vi "G#Object_Deserialize.vi"(0 "reference in":refnum<class "G#Object.lvclass">, 1 "as xml (F)":bool, 2 "serialized object":string, 3 "class attributes (F)":bool, 4 "object id":u32[](array[numeric]), 5 "error in (no error)":errorcluster, 7 "include aggregates (T)":bool=TRUE) -> (14 "reference out":refnum<class "G#Object.lvclass">, 18 "object id out":u32[](array[numeric]), 19 "error out":errorcluster)   [LabVIEW 2020, in "G#Object.lvclass"]
doc: "Deserialize an object from a binary or XML string. \n\nNotice: Deserialization of aggregated objects is not supported by XML."
uses:
  G#Object.lvclass
  utils/G#Object_State.ctl
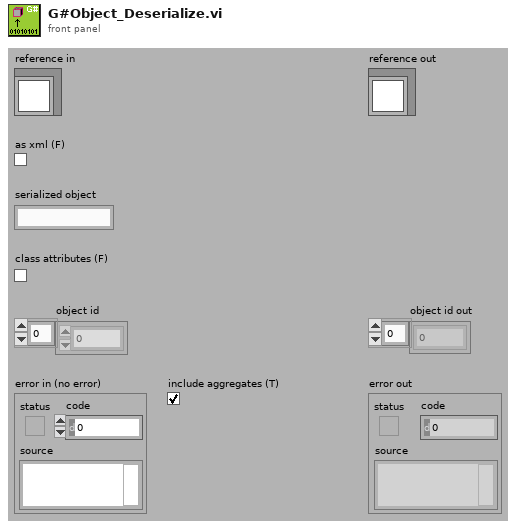
[diagram p1: front panel]
types:
  T1 = typedef "G#Object.lvclass/G#Object_State.ctl" = enum16{"Clear", "Create", "Delete", "Get class attributes", "Class hierarchy", "Get attribute value", "Set attribute value"}
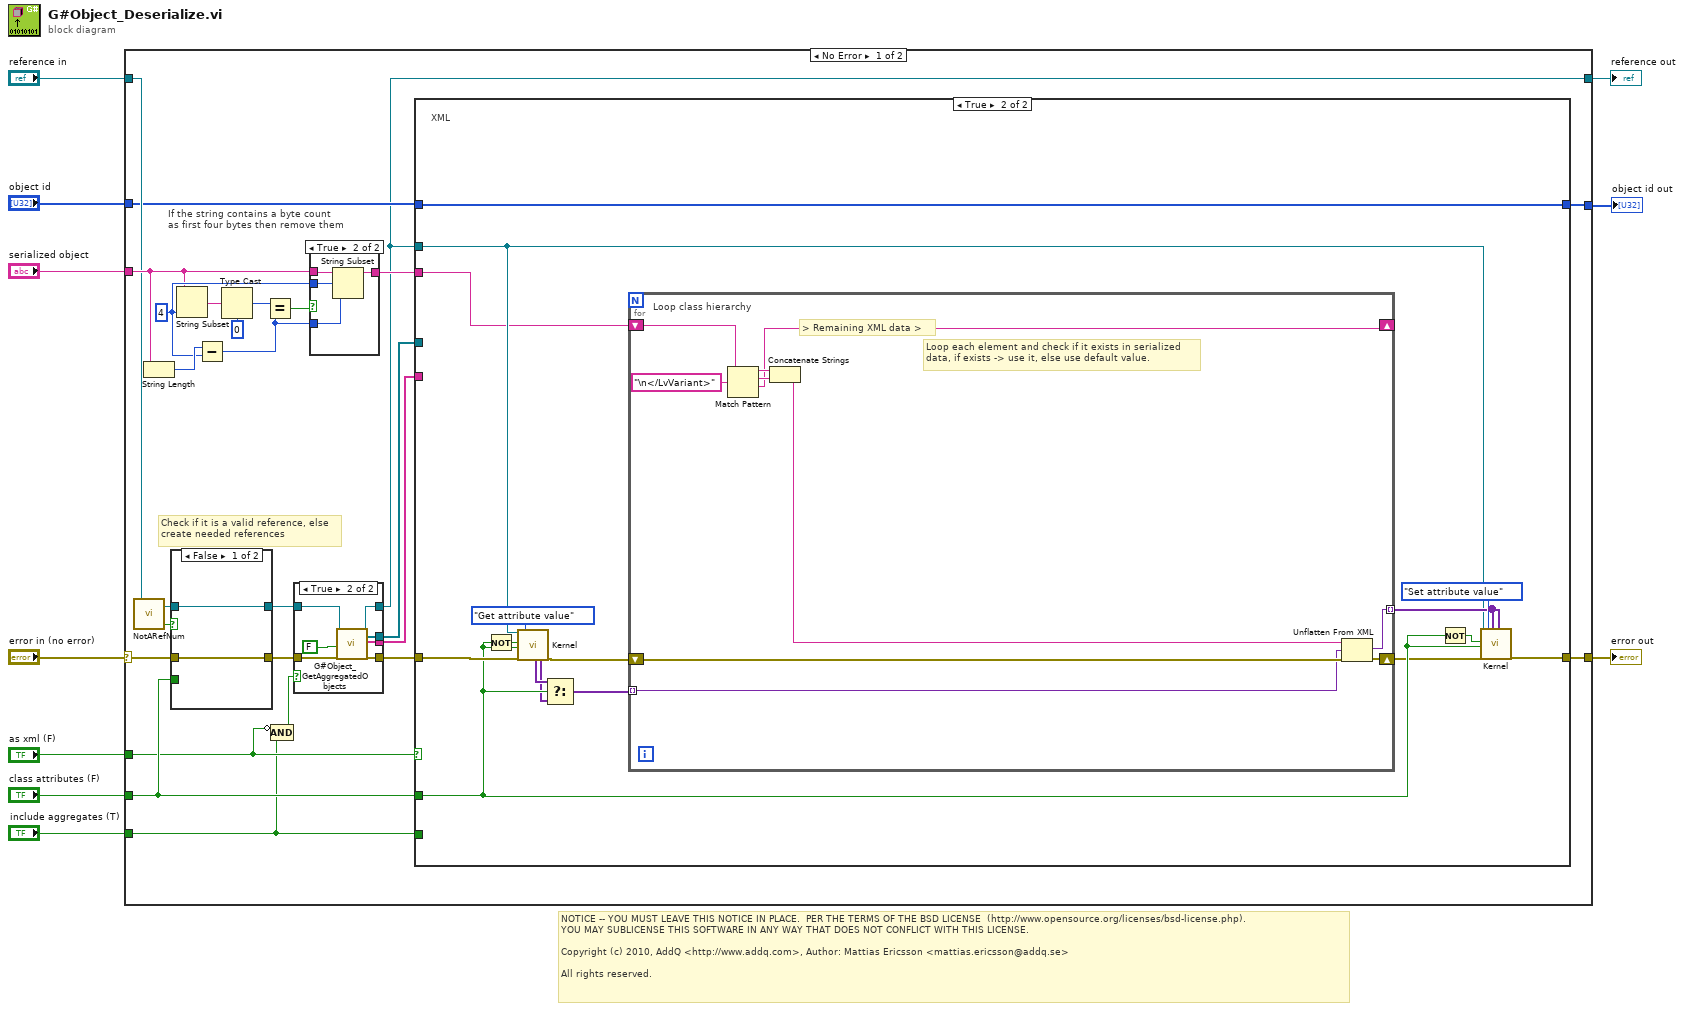
[diagram p0: block diagram]
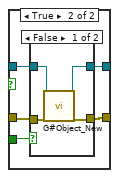
[diagram p3: hidden frame]
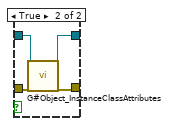
[diagram p4: hidden frame]
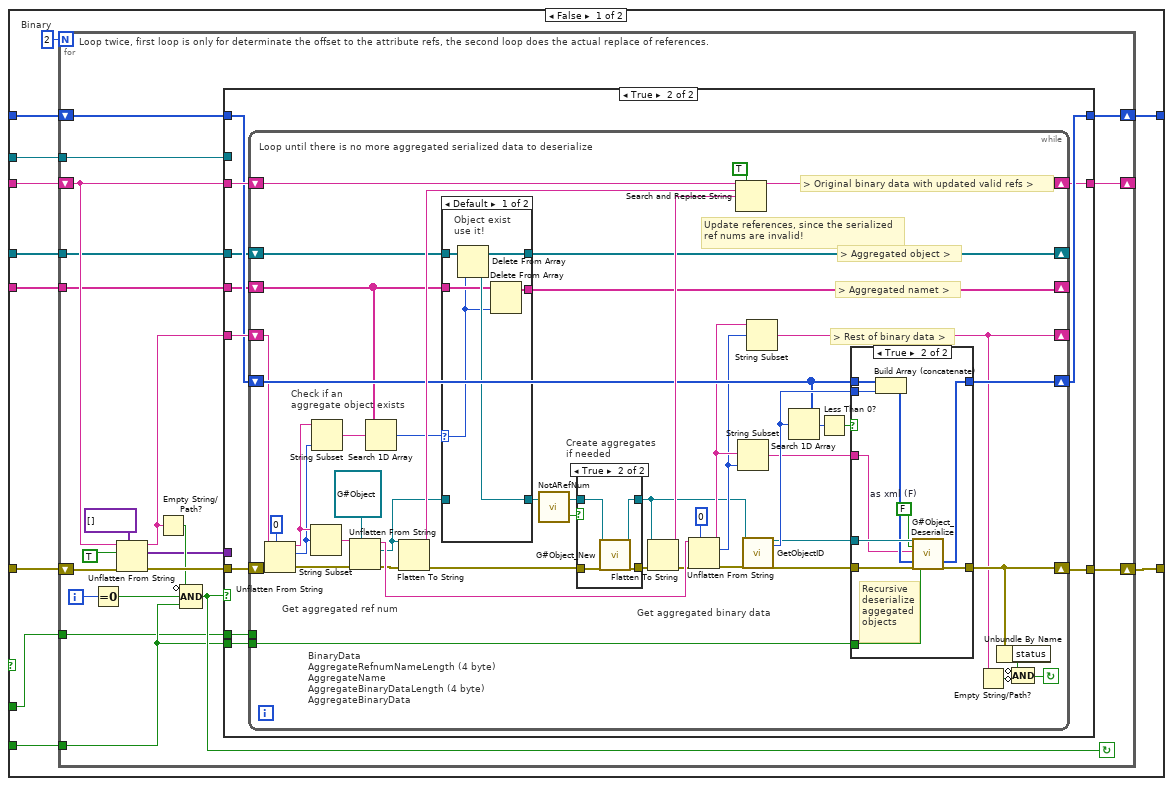
[diagram p6: hidden frame]
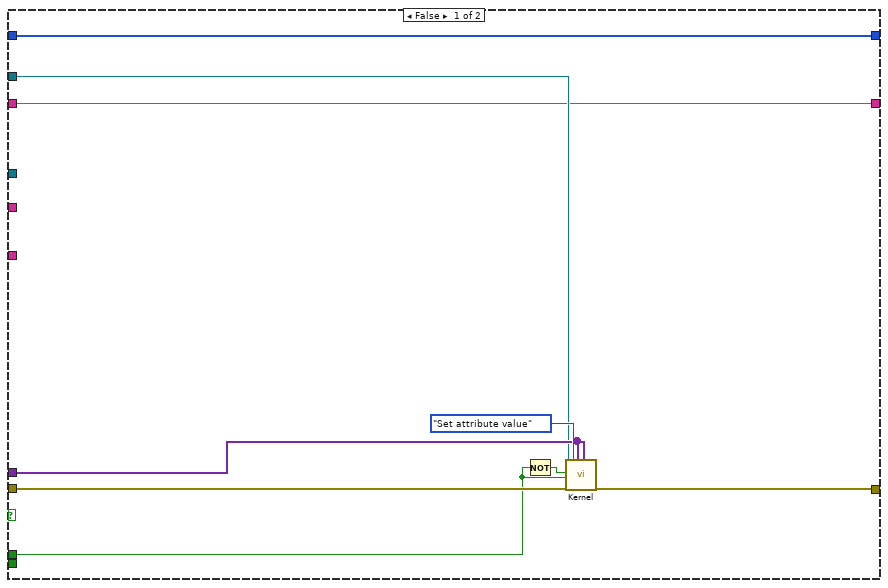
[diagram p7: hidden frame]
diagram:
  # "NOTICE -- YOU MUST LEAVE THIS NOTICE IN PLACE.  PER THE TERMS OF THE BSD LICENSE  (http://www.opensource.org/licenses/bsd-license.php).\nYOU MAY SUBLICENSE THIS SOFTWARE IN ANY WAY THAT DOES NOT CONFLICT WITH THIS LICENSE.\n\nCopyright (c) 2010, AddQ <http://www.addq.com>, Author: Mattias Ericsson <mattias.ericsson@addq.se>\n\nAll rights reserved."
  n1 = case shown="No Error" "error in (no error)" {
    selector: "error in (no error)" -> [w27 w219]
    tunnel: [w22 w219] -> w9
    tunnel: [w17 w218] -> w7
    tunnel: "reference in" -> [w25 w218]
    tunnel: "serialized object" -> [w29 _]
    tunnel: "class attributes (F)" -> [w20 _]
    tunnel: "as xml (F)" -> [w12 _]
    tunnel: "object id" -> [w23 w217]
    tunnel: [w21 w217] -> w2
    tunnel: "include aggregates (T)" -> [w11 _]
    frame No Error {
      w32 = 4 ("length (rest)")
      # "Check if it is a valid reference, else\ncreate needed references"
      # "If the string contains a byte count\nas first four bytes then remove them"
      n2 = call-dynamic "NotARefNum.vi"("reference in"=w25) -> ("not a refnum?"=w24:bool, "reference out"=w26:refnum<class "G#Object.lvclass">)  [unwired: 1 in]
      n3 = String Length(string=w29) -> (length=w36:i32)
      n4 = case shown="False" w24 {
        tunnel: w27 -> [w46 w52]
        tunnel: w20 -> [_ w50]
        tunnel: [w46 w48] -> w19
        tunnel: [w47 w49] -> w18
        tunnel: w26 -> [w47 w51]
        frame False {
        }
        frame True {
          n5 = case shown="False" w50 {
            tunnel: w52 -> [w56 w60]
            tunnel: w51 -> [w55 w59]
            tunnel: [w54 w57] -> w49
            tunnel: [w53 w58] -> w48
            frame False {
              n6 = call "G#Object_New.vi"("reference in"=w55, "error in (no error)"=w56) -> ("reference out"=w54:refnum<class "G#Object.lvclass">, "error out"=w53:errorcluster)  [unwired: 15 in, 1 out]
            }
            frame True {
              n7 = call "G#Object_InstanceClassAttributes.vi"("reference in"=w59, "error in (no error)"=w60) -> ("reference out"=w57:refnum<class "G#Object.lvclass">, "error out"=w58:errorcluster)  [unwired: 14 in, 2 out]
            }
          }
        }
      }
      n8 = String Subset(string=w29, length (rest)=w32) -> (substring=w35:string)  [unwired: 1 in]
      n9 = Subtract(x=w36, y=w32) -> (x-y=w30:i32)
      n10 = Type Cast(type=0, x=w35) -> (*(type *) &x=w33:i32)
      n11 = Equal?(x=w33, y=w30) -> (x = y?=w31:bool)
      n12 = Compound Arithmetic op=AND(invert w12, w11) -> (w13:bool)
      n13 = case shown="True" w13 {
        tunnel: w19 -> [w37 w45]
        tunnel: w18 -> [w38 w44]
        tunnel: [w38 w43] -> w17
        tunnel: [w37 w41] -> w16
        tunnel: [_ w40] -> w15
        tunnel: [_ w39] -> w14
        frame False {
        }
        frame True {
          n14 = call "G#Object_GetAggregatedObjects.vi"("reference in"=w44, "array names (T)"=FALSE, "error in (no error)"=w45) -> ("reference out"=w43:refnum<class "G#Object.lvclass">, "aggregated objects"=w39:refnum<class "G#Object.lvclass">[], "aggregated names"=w40:string[], "error out"=w41:errorcluster)  [unwired: 13 in]
        }
      }
      n15 = case shown="True" w31 {
        tunnel: w29 -> [w61 w65]
        tunnel: [w61 w64] -> w28
        tunnel: w32 -> [_ w63]
        tunnel: w30 -> [_ w62]
        frame False {
        }
        frame True {
          n16 = String Subset(string=w65, offset (0)=w63, length (rest)=w62) -> (substring=w64:string)
        }
      }
      n17 = case shown="True" w12 {
        tunnel: w16 -> [w75 w206]
        tunnel: [w73 w205] -> w22
        tunnel: w28 -> [w76 w192]
        tunnel: w20 -> [w71 w204]
        tunnel: w11 -> [w70 _]
        tunnel: w23 -> [w72 w203]
        tunnel: w17 -> [w68 w193]
        tunnel: [w69 w203] -> w21
        tunnel: w15 -> [w67 _]
        tunnel: w14 -> [w66 _]
        frame False {
          # "Binary"
          n18 = for {
            N: 2 -> [_]
            shift-right: [w92] -> w73
            shift-left: w75 -> [w94]
            shift-right: [w83] -> _
            shift-left: w76 -> [w81]
            shift-right: [w86] -> w69
            shift-left: w72 -> [w87]
            tunnel: w71 -> [w80]
            tunnel: w70 -> [w84]
            tunnel: w68 -> [w79]
            tunnel: w67 -> [w78]
            tunnel: w66 -> [w77]
            i -> [w89]
            stop <- w90 continue-if-true
            # "Loop twice, first loop is only for determinate the offset to the attribute refs, the second loop does the actual replace of references."
            n19 = Equal To 0?(x=w89) -> (x = 0?=w88:bool)
            n20 = Unflatten From String(type=variant[] [] ("first subarray"), binary string=w81, data includes array or string size? (T)=TRUE, error in (no error)=w94) -> (rest of the binary string=w82:string, value=w85:variant[], error out=w93:errorcluster)  [unwired: 1 in]
            n21 = Empty String/Path?(string/path=w82) -> (empty?=w91:bool)
            n22 = Compound Arithmetic op=AND(invert w91, w88, w84) -> (w90:bool)
            n23 = case shown="True" w90 {
              tunnel: w93 -> [w103 w116]
              tunnel: [w102 w111] -> w92
              tunnel: w82 -> [_ w115]
              tunnel: w81 -> [w97 w114]
              tunnel: w87 -> [w99 w113]
              tunnel: [w99 w112] -> w86
              tunnel: w85 -> [w101 _]
              tunnel: w80 -> [w100 w110]
              tunnel: w79 -> [w98 _]
              tunnel: w84 -> [_ w109]
              tunnel: [w97 w108] -> w83
              tunnel: w78 -> [_ w107]
              tunnel: w77 -> [_ w106]
              frame False {
                n24 = Not(x=w100) -> (.not. x?=w105:bool)
                n25 = call-dynamic "Kernel.vi"("reference in"=w98, "option 1"=w105, "option 2"=w100, "error in (no error)"=w103, "state"=G#Object_State."Set attribute value" ("State"), "attributes in"=w101, "class attributes in"=w101) -> ("error out"=w102:errorcluster)  [unwired: 4 in, 8 out]
              }
              frame True {
                n26 = while {
                  shift-right: [w134] -> _
                  shift-left: w115 -> [w142]
                  shift-right: [w137] -> w111
                  shift-left: w116 -> [w144]
                  shift-right: [w159] -> w108
                  shift-left: w114 -> [w162]
                  shift-right: [w153] -> w112
                  shift-left: w113 -> [w154]
                  tunnel: w110 -> [_]
                  tunnel: w109 -> [w151]
                  shift-right: [w119] -> _
                  shift-left: w106 -> [w120]
                  shift-right: [w117] -> _
                  shift-left: w107 -> [w118]
                  stop <- w135 continue-if-true
                  # "> Original binary data with updated valid refs >"
                  # "> Rest of binary data >"
                  # "> Aggregated namet >"
                  # "> Aggregated object >"
                  # "Loop until there is no more aggregated serialized data to deserialize"
                  # "Get aggregated binary data"
                  # "Get aggregated ref num"
                  # "Check if an\naggregate object exists"
                  # "Create aggregates\nif needed"
                  # "BinaryData\nAggregateRefnumNameLength (4 byte)\nAggregateName\nAggregateBinaryDataLength (4 byte)\nAggregateBinaryData"
                  # "Update references, since the serialized\nref nums are invalid!"
                  n27 = Unflatten From String(type=0 ("length"), binary string=w142, error in (no error)=w144) -> (rest of the binary string=w139:string, value=w138:i32, error out=w143:errorcluster)  [unwired: 2 in]
                  n28 = String Subset(string=w139, offset (0)=w138) -> (substring=w140:string)  [unwired: 1 in]
                  n29 = String Subset(string=w139, length (rest)=w138) -> (substring=w124:string)  [unwired: 1 in]
                  n30 = Unflatten From String(type=refnum<class "G#Object.lvclass"> refnum ("G#Object.lvclass"), binary string=w140, error in (no error)=w143) -> (rest of the binary string=w149:string, value=w121:refnum<class "G#Object.lvclass">, error out=w132:errorcluster)  [unwired: 2 in]
                  n31 = Search 1D Array(1D array=w118, element=w124) -> (index of element=w123:i32)  [unwired: 1 in]
                  n32 = Flatten To String(anything=w121, error in (no error)=w132) -> (data string=w160:string, error out=w125:errorcluster)  [unwired: 2 in, 1 out]
                  n33 = case shown="Default" w123 {
                    selector: w123 -> [w164 _]
                    tunnel: w121 -> [_ w172]
                    tunnel: [w168 w172] -> w122
                    tunnel: w120 -> [w169 w171]
                    tunnel: [w167 w171] -> w119
                    tunnel: w118 -> [w166 w170]
                    tunnel: [w165 w170] -> w117
                    frame Default {
                      # "Object exist\nuse it!"
                      n34 = Delete From Array(array=w169, index=w164) -> (deleted portion=w168:refnum<class "G#Object.lvclass">, array with subset deleted=w167:refnum<class "G#Object.lvclass">[])  [unwired: 1 in]
                      n35 = Delete From Array(array=w166, index=w164) -> (array with subset deleted=w165:string[])  [unwired: 1 in, 1 out]
                    }
                    frame -1 {
                    }
                  }
                  n36 = call-dynamic "NotARefNum.vi"("reference in"=w122) -> ("not a refnum?"=w131:bool, "reference out"=w129:refnum<class "G#Object.lvclass">)  [unwired: 1 in]
                  n37 = case shown="True" w131 {
                    tunnel: w125 -> [w174 w178]
                    tunnel: [w174 w177] -> w130
                    tunnel: w129 -> [w173 w176]
                    tunnel: [w173 w175] -> w128
                    frame False {
                    }
                    frame True {
                      n38 = call "G#Object_New.vi"("reference in"=w176, "error in (no error)"=w178) -> ("reference out"=w175:refnum<class "G#Object.lvclass">, "error out"=w177:errorcluster)  [unwired: 15 in, 1 out]
                    }
                  }
                  n39 = Flatten To String(anything=w128, error in (no error)=w130) -> (data string=w161:string, error out=w127:errorcluster)  [unwired: 2 in, 1 out]
                  n40 = Unflatten From String(type=0 ("length"), binary string=w149, error in (no error)=w127) -> (rest of the binary string=w146:string, value=w145:i32, error out=w150:errorcluster)  [unwired: 2 in]
                  n41 = Search and Replace String(replace all?=TRUE ("replace all? (F)"), input string=w162, search string=w160, replace string=w161) -> (result string=w159:string)  [unwired: 4 in, 3 out]
                  n42 = String Subset(string=w146, length (rest)=w145) -> (substring=w147:string)  [unwired: 1 in]
                  n43 = call-dynamic "GetObjectID.vi"("reference in"=w128, "error in (no error)"=w150) -> ("reference out"=w157:refnum<class "G#Object.lvclass">, "object ID"=w158:u32, "error out"=w156:errorcluster)  [unwired: 15 in]
                  n44 = String Subset(string=w146, offset (0)=w145) -> (substring=w134:string)  [unwired: 1 in]
                  n45 = Search 1D Array(1D array=w154, element=w158) -> (index of element=w155:i32)  [unwired: 1 in]
                  n46 = Less Than 0?(x=w155) -> (x < 0?=w152:bool)
                  n47 = case shown="True" w152 {
                    tunnel: w158 -> [_ w190]
                    tunnel: w157 -> [_ w189]
                    tunnel: w156 -> [w179 w188]
                    tunnel: w154 -> [w180 w187]
                    tunnel: [w180 w186] -> w153
                    tunnel: [w179 w184] -> w137
                    tunnel: w147 -> [_ w183]
                    tunnel: w151 -> [_ w181]
                    frame False {
                      # "Do not deserialize\na dead or already\ndeserialized object"
                    }
                    frame True {
                      w182 = FALSE  # as xml (F)
                      # "Recursive\ndeserialize\naggegated\nobjects"
                      n48 = Build Array (concatenate)(w187, w190) -> (w185:u32[])
                      n49 = call-dynamic "G#Object_Deserialize.vi"("reference in"=w189, "as xml (F)"=w182, "serialized object"=w183, "object id"=w185, "error in (no error)"=w188, "include aggregates (T)"=w181) -> ("object id out"=w186:u32[], "error out"=w184:errorcluster)  [unwired: 11 in, 1 out]
                    }
                  }
                  n50 = Empty String/Path?(string/path=w134) -> (empty?=w133:bool)
                  n51 = Unbundle By Name(w137) -> ("status"=w136:bool)
                  n52 = Compound Arithmetic op=AND(invert w136, invert w133) -> (w135:bool)
                }
              }
            }
          }
        }
        frame True {
          # "XML"
          n53 = Not(x=w204) -> (.not. x?=w199:bool)
          n54 = call-dynamic "Kernel.vi"("reference in"=w193, "option 1"=w199, "option 2"=w204, "error in (no error)"=w206, "state"=G#Object_State."Get attribute value" ("State")) -> ("class attributes out"=w201:variant[], "attributes out"=w200:variant[], "error out"=w191:errorcluster)  [unwired: 6 in, 6 out]
          n55 = Select(t=w201, s=w204, f=w200) -> (s? t:f=w198:variant[])
          n56 = for {
            tunnel: w198 -> [w209] mode=indexing
            tunnel: [w215] -> w194 mode=indexing
            shift-right: [w216] -> w195
            shift-left: w191 -> [w210]
            shift-right: [w207] -> _
            shift-left: w192 -> [w214]
            # "> Remaining XML data >"
            # "Loop class hierarchy"
            # "Loop each element and check if it exists in serialized\ndata, if exists -> use it, else use default value."
            n57 = Match Pattern(string=w214, regular expression="\n</LvVariant>") -> (before substring=w212:string, match substring=w211:string, after substring=w207:string)  [unwired: 1 in, 1 out]
            n58 = Concatenate Strings(w212, w211) -> (w208:string)
            n59 = Unflatten From XML(xml string=w208, type=w209, error in (no error)=w210) -> (value=w215:variant, error out=w216:errorcluster)
          }
          n60 = Not(x=w204) -> (.not. x?=w197:bool)
          n61 = call-dynamic "Kernel.vi"("reference in"=w193, "option 1"=w197, "option 2"=w204, "error in (no error)"=w195, "state"=G#Object_State."Set attribute value" ("State"), "attributes in"=w194, "class attributes in"=w194) -> ("error out"=w205:errorcluster)  [unwired: 4 in, 8 out]
        }
      }
    }
    frame Error {
    }
  }
  "error out" <- w9
  "reference out" <- w7
  "object id out" <- w2
